vi "settings tester.vi"() -> ()   [LabVIEW 2021]
panel:
  in  "Write":T1={"baud rate"=115200, "data bits"=8, "parity"=enum."None", "stop bits"=10, "flow control"=enum."None", "delay"=50} {"stop bits" items=["1.0"=10, "1.5"=15, "2.0"=20]; "baud rate" max=921600; "data bits" max=16}
  out "Read":T1={"baud rate"=115200, "data bits"=8, "parity"=enum."None", "stop bits"=10, "flow control"=enum."None", "delay"=50} {"stop bits" items=["1.0"=10, "1.5"=15, "2.0"=20]; "baud rate" max=921600; "data bits" max=16}
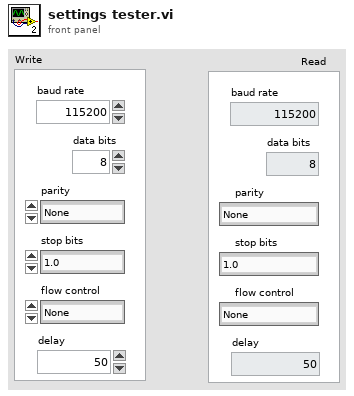
[diagram p1: front panel]
types:
  T1 = cluster{"baud rate":u32, "data bits":u8, "parity":enum16{"None", "Odd", "Even", "Mark", "Space"}, "stop bits":u16, "flow control":enum16{"None", "XON/XOFF", "RTS/CTS", "DTR/DSR"}, "delay":u16}
  T2 = cluster{"COM":refnum<visa-resource-name>, "baud rate":u32, "data bits":u8, "parity":enum16{"None", "Odd", "Even", "Mark", "Space"}, "stop bits":u16, "flow control":enum16{"None", "XON/XOFF", "RTS/CTS", "DTR/DSR"}, "delay":u16}
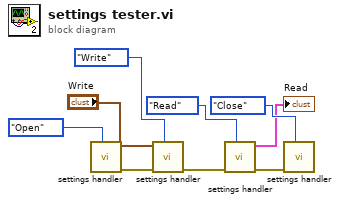
[diagram p0: block diagram]
diagram:
  n1 = call "settings handler.vi"("Operation"=enum16{"Open", "Write", "Read", "Close"}."Open") -> ("Error Out"=w5:errorcluster)  [unwired: 8 in, 2 out]
  n2 = call "settings handler.vi"("Operation"=enum16{"Open", "Write", "Read", "Close"}."Write", "error in (no error)"=w5, "Write"="Write") -> ("Error Out"=w4:errorcluster)  [unwired: 6 in, 2 out]
  n3 = call "settings handler.vi"("Operation"=enum16{"Open", "Write", "Read", "Close"}."Read", "error in (no error)"=w4) -> ("Error Out"=w3:errorcluster, "Read"=→"Read":T2)  [unwired: 7 in, 1 out]
  n4 = call "settings handler.vi"("Operation"=enum16{"Open", "Write", "Read", "Close"}."Close", "error in (no error)"=w3) -> ()  [unwired: 7 in, 3 out]
